vi "Event handler-Update AOL globals on UI events.vi"(8 "error in (no error)":errorcluster) -> (0 "error out":errorcluster)   [LabVIEW 2013]
uses:
  Global Variables/gl_UI Ctrl Refs.vi
  Global Variables/General Globals.vi
  Configuration code/Calibration/Globals/gl_Calibration globals.vi
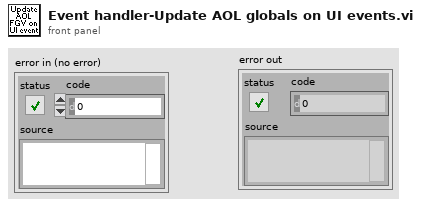
[diagram p1: front panel]
types:
  T1 = typedef "UI ctrl refs cluster.ctl" = cluster{"Top level VI path":path, "Top level VI ref":refnum<vi>, "User menu ref":refnum<k9>, "Sub Panel control":refnum<vi>, "Imaging Param Tab":refnum<vi>, "Occurrence-Start drivers":refnum<k4>, "Occurrence-Speed logging initialised":refnum<k4>, "Occurrence-XYZ stage initialised":refnum<k4>, "Exit button":refnum<vi>, "Status ind":refnum<vi>, "Return to Origin":refnum<vi>, "Speed Logging":refnum<vi>, "Time Lapse":refnum<vi>, "Live Imaging":refnum<vi>, "AOL Z Stack":refnum<vi>, "Motor Z Stack":refnum<vi>, "Funct Acq button":refnum<vi>, "Hard Shutter":refnum<vi>, "Virtual Shutter":refnum<vi>, "Laser Power":refnum<vi>, "AOL Mode":refnum<vi>, "Frame Size":refnum<vi>, "Field of View":refnum<vi>, "Dwell Time":refnum<vi>, "Zoom":refnum<vi>, "AOL Z":refnum<vi>, "Objective":refnum<vi>, "Axis":refnum<vi>, "Paths & Names":refnum<vi>, "Experiment folder path (ind.)":refnum<vi>, "Last State (Ind.)":refnum<vi>, "Laser wavelength ind (nm)":refnum<vi>, "Averages":refnum<vi>, "Angle (degrees)":refnum<vi>, "X centre":refnum<vi>, "Y centre":refnum<vi>, "Plane Mode":refnum<vi>, "# Planes":refnum<vi>, "Z Start":refnum<vi>, "Z Stop":refnum<vi>, "Z Step":refnum<vi>, "PMT 1":refnum<vi>, "PMT 2":refnum<vi>, "Stage XYZ Position":refnum<vi>, "Pockels@Z Start":refnum<vi>, "Pockels@Z Stop":refnum<vi>, "Obtain Z Start":refnum<vi>, "Obtain Z Stop":refnum<vi>, "Live stim.trig.period":refnum<vi>, "Live stim.trig.enable":refnum<vi>, "Funct. Acq. Pockels Modulation":refnum<vi>, "Enable Video Recording":refnum<vi>, "Video Record-Live Imaging":refnum<vi>, "Video Record-Funct acq":refnum<vi>, "AOL Z-stack Chirps Ready (ind)":refnum<vi>, "Center freq ind (nm)":refnum<vi>, "Logging queue (ind)":refnum<vi>, "Back aperture power (ind.)":refnum<vi>, "Power after objective (ind.)":refnum<vi>, "Switch user":refnum<vi>}
  T2 = typedef "Laser control knob.ctl" = u16
  T3 = typedef "AOL modes.ctl" = enum16{"Raster", "Structural", "Pointing", "Mini Scan", "Alignment"}
  T4 = typedef "Plane Mode.ctl" = u16
  T5 = typedef "AOL_Globals.ctl" = cluster{"Imaging Protocol":T6, "Number of POI":u16, "Number of Miniscans":u16, "Number of Trials":u16, "Number of Cycles ":u64, "# Averaged Frames":u16, "Laser power (%)":u8, "Pockels":dbl, "Acquisition Length (sec)":dbl, "Fill time (us)":dbl, "POI Dwell time (us)":dbl, "Miniscan Dwell time per pixel (us)":dbl, "PMT 1":dbl, "PMT 2":dbl, "Back Apperture":dbl, "Frame Size":T7, "Center Frequency":dbl, "Field of View":dbl, "DwellTime (us)":dbl, "Wavelength (nm)":dbl, "Zoom":dbl, "AOL Z":dbl, "AOL Mode":T3, "GridXY":dbl, "GridZ":dbl, "TriggerPeriod (sec)":dbl, "Number of Pixels in Miniscan":u16, "Experiment folder path":path, "X centre":dbl, "Y centre":dbl, "Angle (degrees)":dbl, "Plane Mode":T4, "Threshold":u16[], "Regenerate Chirps":bool, "Rectangle ROI length (pixels)":u16, "Rectangle ROI height (pixels)":u16, "AOD fill":u16, "Samples Wait after Trigger":u16, "StartUp Delay":i32, "Slip Cycle":u32, "Add Cycle":bool}
  T6 = typedef "Imaging Protocols enum.ctl" = enum16{"AOL Z-Stack", "Motor Z Stack", "Functional Acquisition", "Single Plane Acquisition", "Volume Acquisition", "Live Imaging", "Live Plane Imaging", "Live Volume Imaging"}
  T7 = typedef "Frame Size.ctl" = u16
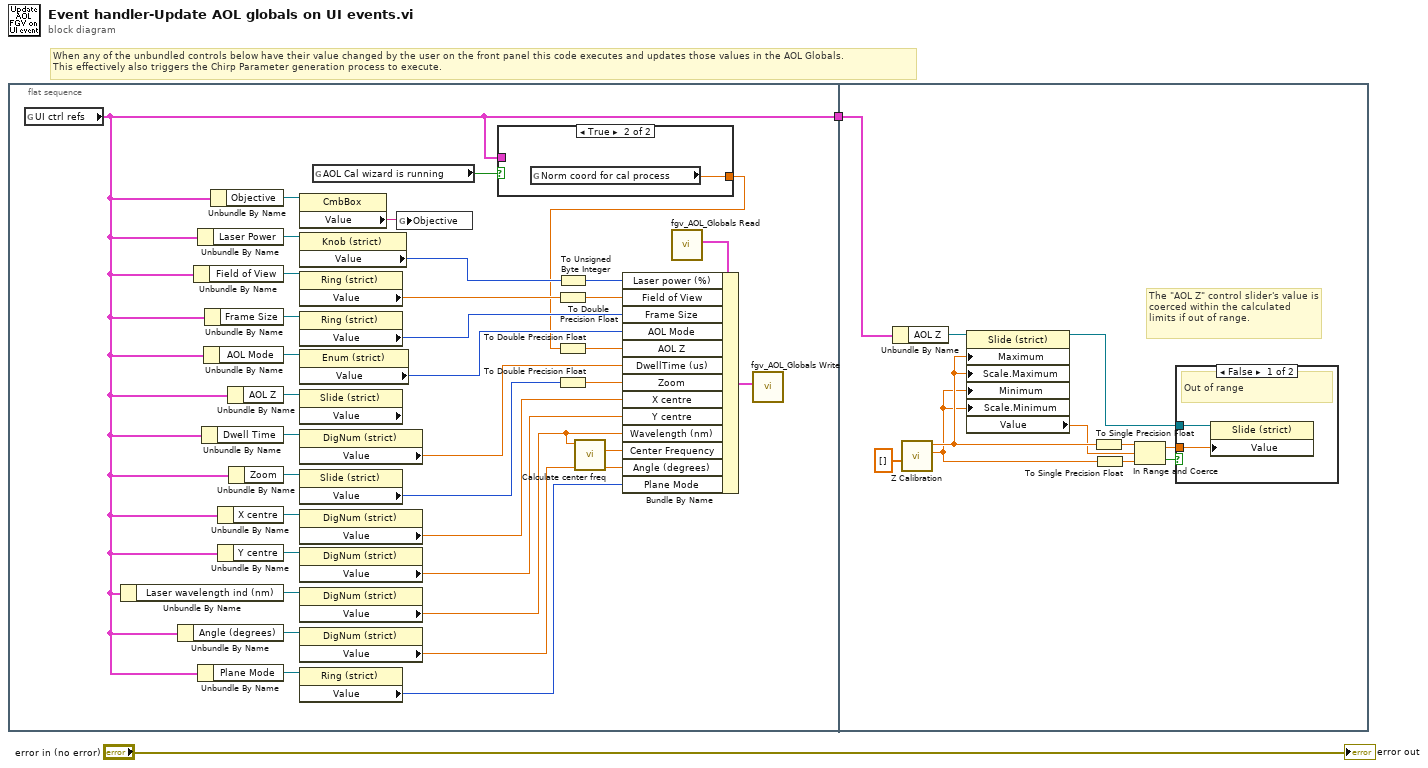
[diagram p0: block diagram]
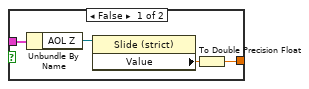
[diagram p2: hidden frame]
diagram:
  # "When any of the unbundled controls below have their value changed by the user on the front panel this code executes and updates those values in the AOL Globals.\nThis effectively also triggers the Chirp Parameter generation process to execute."
  n1 = flat-sequence {
    tunnel: [w5] -> w2
    tunnel: w2 -> [w46]
    frame #0 {
      n2 = global read "gl_UI Ctrl Refs.vi" "UI ctrl refs"() -> (w5:T1)
      n3 = Unbundle By Name(w5) -> ("Laser wavelength ind (nm)"=w18:refnum<vi>)
      n4 = Unbundle By Name(w5) -> ("Angle (degrees)"=w19:refnum<vi>)
      n5 = Unbundle By Name(w5) -> ("Field of View"=w34:refnum<vi>)
      n6 = Unbundle By Name(w5) -> ("Laser Power"=w35:refnum<vi>)
      n7 = Unbundle By Name(w5) -> ("Plane Mode"=w20:refnum<vi>)
      n8 = Unbundle By Name(w5) -> ("Dwell Time"=w30:refnum<vi>)
      n9 = Unbundle By Name(w5) -> ("AOL Mode"=w32:refnum<vi>)
      n10 = Unbundle By Name(w5) -> ("Frame Size"=w33:refnum<vi>)
      n11 = Unbundle By Name(w5) -> ("Objective"=w24:refnum<vi>)
      n12 = Unbundle By Name(w5) -> ("X centre"=w16:refnum<vi>)
      n13 = Unbundle By Name(w5) -> ("Y centre"=w17:refnum<vi>)
      n14 = Unbundle By Name(w5) -> ("AOL Z"=w31:refnum<vi>)
      n15 = Unbundle By Name(w5) -> ("Zoom"=w29:refnum<vi>)
      n16 = property class="CmbBox"(reference=w24) -> ("Value"=w22:string)  [unwired: 1 in, 2 out]
      n17 = property class="Knob (strict)"(reference=w35) -> ("Value"=w28:T2)  [unwired: 1 in, 2 out]
      n18 = property class="Ring (strict)"(reference=w34) -> ("Value"=w23:sgl)  [unwired: 1 in, 2 out]
      n19 = property class="Ring (strict)"(reference=w33) -> ("Value"=w8:u16)  [unwired: 1 in, 2 out]
      n20 = property class="Enum (strict)"(reference=w32) -> ("Value"=w27:T3)  [unwired: 1 in, 2 out]
      n21 = property class="Slide (strict)" props=["Value"](reference=w31) -> ()  [unwired: 1 in, 3 out]
      n22 = property class="DigNum (strict)"(reference=w30) -> ("Value"=w26:dbl)  [unwired: 1 in, 2 out]
      n23 = property class="Slide (strict)"(reference=w29) -> ("Value"=w25:i8)  [unwired: 1 in, 2 out]
      n24 = property class="DigNum (strict)"(reference=w16) -> ("Value"=w15:dbl)  [unwired: 1 in, 2 out]
      n25 = property class="DigNum (strict)"(reference=w17) -> ("Value"=w14:dbl)  [unwired: 1 in, 2 out]
      n26 = property class="DigNum (strict)"(reference=w18) -> ("Value"=w3:dbl)  [unwired: 1 in, 2 out]
      n27 = property class="DigNum (strict)"(reference=w19) -> ("Value"=w13:dbl)  [unwired: 1 in, 2 out]
      n28 = property class="Ring (strict)"(reference=w20) -> ("Value"=w12:T4)  [unwired: 1 in, 2 out]
      n29 = global read "gl_Calibration globals.vi" "AOL Cal wizard is running"() -> (w7:bool)
      n30 = global write "General Globals.vi" "Objective"(w22) -> ()
      n31 = case shown="True" w7 {
        tunnel: [w39 w42] -> w6
        tunnel: w5 -> [w38 _]
        frame False {
          n32 = Unbundle By Name(w38) -> ("AOL Z"=w41:refnum<vi>)
          n33 = property class="Slide (strict)"(reference=w41) -> ("Value"=w40:sgl)  [unwired: 1 in, 2 out]
          n34 = To Double Precision Float(number=w40) -> (double precision float=w39:dbl)
        }
        frame True {
          n35 = global read "gl_Calibration globals.vi" "Norm coord for cal process"() -> (w42:dbl)
        }
      }
      n36 = To Unsigned Byte Integer(number=w28) -> (unsigned 8bit integer=w9:u8)
      n37 = To Double Precision Float(number=w23) -> (double precision float=w10:dbl)
      n38 = To Double Precision Float(number=w6) -> (double precision float=w11:dbl)
      n39 = To Double Precision Float(number=w25) -> (double precision float=w21:dbl)
      n40 = call "Calculate center freq.vi"("UI Wavelength"=w3) -> ("Centre frequency (MHz)"=w4:dbl)  [unwired: 9 in, 1 out]
      n41 = call "fgv_AOL_Globals Read.vi"() -> ("AOL_Globals"=w37:T5)  [unwired: 9 in, 2 out]
      n42 = Bundle By Name(cluster=w37, "Laser power (%)"=w9, "Field of View"=w10, "Frame Size"=w8, "AOL Mode"=w27, "AOL Z"=w11, "DwellTime (us)"=w26, "Zoom"=w21, "X centre"=w15, "Y centre"=w14, "Wavelength (nm)"=w3, "Center Frequency"=w4, "Angle (degrees)"=w13, "Plane Mode"=w12) -> (w36:T5)
      n43 = call "fgv_AOL_Globals Write.vi"("AOL_Globals"=w36) -> ()  [unwired: 10 in, 1 out]
    }
    frame #1 {
      # "The \"AOL Z\" control slider's value is coerced within the calculated limits if out of range."
      n44 = Unbundle By Name(w46) -> ("AOL Z"=w45:refnum<vi>)
      n45 = call "Z Calibration.vi"("Z Planes"=dbl[] [] ("Motor Z")) -> ("Z Min"=w44:dbl, "Z Max"=w52:dbl)  [unwired: 7 in, 2 out]
      n46 = property on="Property Node" class="Slide (strict)"(reference=w45, "Maximum"=w52, "Scale.Maximum"=w52, "Minimum"=w44, "Scale.Minimum"=w44) -> (reference out=w43:refnum<vi>, "Value"=w51:sgl)  [unwired: 1 in, 1 out]
      n47 = To Single Precision Float(number=w52) -> (single precision float=w50:sgl)
      n48 = To Single Precision Float(number=w44) -> (single precision float=w49:sgl)
      n49 = In Range and Coerce(upper limit=w50, x=w51, lower limit=w49) -> (coerced(x)=w47:sgl, In Range?=w48:bool)
      n50 = case shown="False" w48 {
        tunnel: w47 -> [w55 _]
        tunnel: w43 -> [w54 _]
        frame False {
          # "Out of range"
          n51 = property on="Property Node" class="Slide (strict)"(reference=w54, "Value"=w55) -> ()  [unwired: 1 in, 2 out]
        }
        frame True {
          # "In range"
        }
      }
    }
  }
  "error out" <- "error in (no error)"
